vi "Varian_PUMP_POWER.vi"(8 "error in (no error)":errorcluster, 11 "VISA Refnum in":refnum<visa-resource-name>) -> (0 "error out":errorcluster, 2 "Numeric":dbl, 3 "VISA Refnum out":refnum<visa-resource-name>)   [LabVIEW 2015]
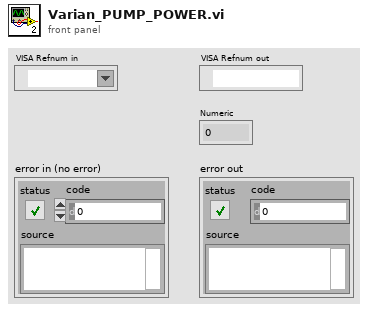
[diagram p1: front panel]
types:
  T1 = enum16{"START", "STOP", "REMOTE/SERIAL", "REMOTE", "SERIAL", "START/STOP", "PUMP STATUS", "Driving Frequency", "PUMP POWER", "PRESSURE"}
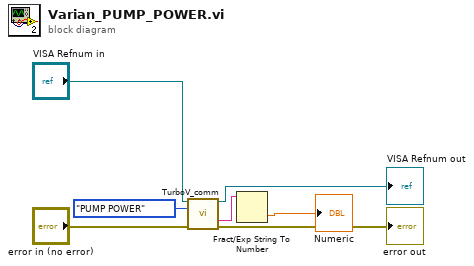
[diagram p0: block diagram]
diagram:
  n1 = call "TurboV_comm.vi"("VISA resource name"="VISA Refnum in", "Command"=T1."PUMP POWER", "error in (no error)"="error in (no error)") -> ("VISA resource name out"=→"VISA Refnum out":refnum<visa-resource-name>, "read buffer"=w6:string, "error out"=→"error out":errorcluster)  [unwired: 10 in]
  n2 = Fract/Exp String To Number(string=w6) -> (number=→"Numeric":dbl)  [unwired: 3 in, 1 out]
